vi "Search element.vi"(8 "error":errorcluster, 9 "element":string, 10 "Colum":i32, 11 "all data":string[][](array[string])) -> (0 "error out":errorcluster, 1 "row data":string[](array[string]), 2 "Status":bool, 3 "index":i32)   [LabVIEW 2017]
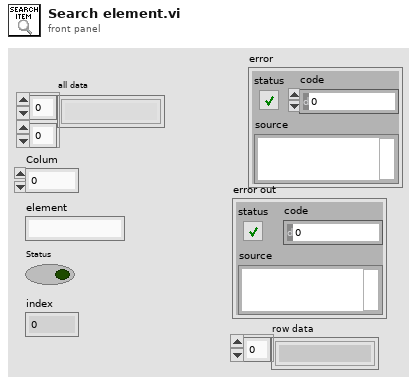
[diagram p1: front panel]
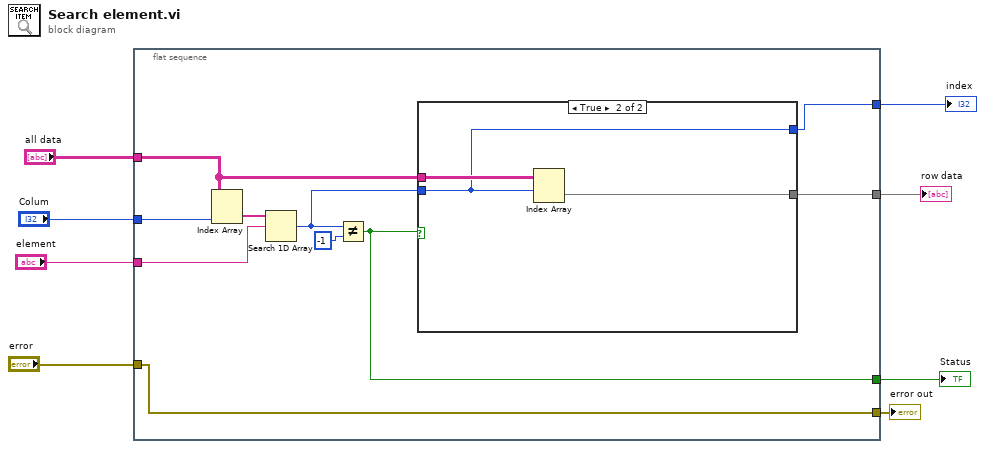
[diagram p0: block diagram]
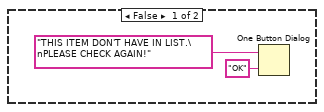
[diagram p2: hidden frame]
diagram:
  n1 = flat-sequence {
    tunnel: [w9] -> w8
    tunnel: [w17] -> w7
    tunnel: "all data" -> [w11]
    tunnel: "Colum" -> [w16]
    tunnel: "element" -> [w14]
    tunnel: "error" -> [w12]
    tunnel: [w12] -> w2
    tunnel: [w10] -> w1
    frame #0 {
      n2 = Index Array "Index Array"(array=w11, index (col)=w16) -> (element=w15:string[])  [unwired: 1 in]
      n3 = Search 1D Array(1D array=w15, element=w14) -> (index of element=w18:i32)  [unwired: 1 in]
      n4 = Not Equal?(x=w18, y=-1) -> (x != y?=w17:bool)
      n5 = case shown="True" w17 {
        tunnel: w18 -> [_ w21]
        tunnel: w11 -> [_ w23]
        tunnel: [_ w22] -> w10
        tunnel: [_ w21] -> w9
        frame False {
          n6 = One Button Dialog(message="THIS ITEM DON'T HAVE IN LIST.\nPLEASE CHECK AGAIN!", button name ("OK")="OK") -> ()  [unwired: 1 out]
        }
        frame True {
          n7 = Index Array "Index Array"(array=w23, index (row)=w21) -> (element=w22:string[])  [unwired: 1 in]
        }
      }
    }
  }
  "index" <- w8
  "Status" <- w7
  "error out" <- w2
  "row data" <- w1
